vi "Acquisition_PharaGlow.vi"() -> ()   [LabVIEW 2021]
uses:
  <vilib>/userdefined/High Color/IMAQdx.ctl
  <vilib>/vision/Image Controls.llb/IMAQ Image.ctl
  <vilib>/vision/driver/IMAQdx.llb/IMAQdx Buffer Number Mode.ctl
  <vilib>/Utility/file.llb/Write Delimited Spreadsheet (string).vi
  <vilib>/Utility/file.llb/Write Delimited Spreadsheet (DBL).vi
  <vilib>/vision/driver/NI_Vision_Acquisition_Software.lvlib
  <resource>/objmgr/imaqdx.rc
  <vilib>/vision/NI_Vision_Development_Module.lvlib
panel:
  in  "Data saving folder":path=path "C:/DefaultFolder/BASLER"
  in  "Choose camera":T1="cam1"
  out "WormCounter":u64
  out "Objects":T2(array[cluster]) {"Aspect Ratio" format="%.2f"; "Orientation" format="%.2f"; "Area" format="%.2f"; "Object Center"."Y" format="%.2f"; "Object Center"."X" format="%.2f"}
  in  "Settings segmentation":T3={"Objects"=0, "Threshold"=24, "Reject Border"=TRUE, "Fill Holes"=FALSE, "Min Object Size"=TRUE, "Min Size"=300, "Max Object Size"=FALSE, "Max Size"=100, "Show Search Area"=FALSE, "Show Center"=FALSE, "Show Bounding Box"=FALSE} {"Objects" items=["Bright Objects", "Dark Objects"]; "Threshold" min=1 max=999999999 step=1; "Max Size" min=1 max=999999999 step=1; "Min Size" min=1 max=999999999 step=1}
  in  "Header Info":string[][](array[string])=[["Frame", "X_left", "Y_top", "X_center", "Y_center", "File_name"]]
  out "Path csv":path
  out "Rec_folder":path
  in  "Segment Data":bool
  out "Im_OneWorm":T4
  out "Im_Segm.":T4
  in  "Image format":string(combo)=".tiff"
  out "Init":bool
  in  "Load settings":bool
  out "Buffer overflow":string
  out "Overflow":bool=TRUE
  out "Buffer used (frames)":u64(slide) scale=0.0..167.0
  out "Expected Time (s)":dbl
  out "RAM needed (GB)":dbl
  out "Time log (ms)":dbl[](array[numeric]) format="%#_14g"
  out "Timestamp":dbl[](array[numeric])
  in  "Camera Control":T5={"Acquisition Freq"=30.0, "Exposure (ms)"=4.0, "Gain"=24.0, "Height"=2064, "Width"=3088, "Acq. trigger start"=FALSE} {"Acquisition Freq" min=1e-06 max=60.0; "Height" min=400 max=2064 step=1; "Width" min=400 max=3088 step=1}
  out "Camera Control copy":T5
  out "All Image Buffers":T4[](array[typedef])
  out "Image Out":T4(plugin-control)
  out "Lost frames":u32
  out "Approx. Frame Rate":dbl
  out "Saved frames":u32
  in  "Acquire button":bool
  in  "Focus button":bool
  out "Readout frames":i32
  in  "Stop":bool caption="Stop (F)"
  out "Finished acquisition":bool=TRUE
  in  "Num frames":u32=2000
  out "#Frames Buffer":u32=4000
  out "Camera Session":T1
  out "Camera config":string
  # "Compact data"
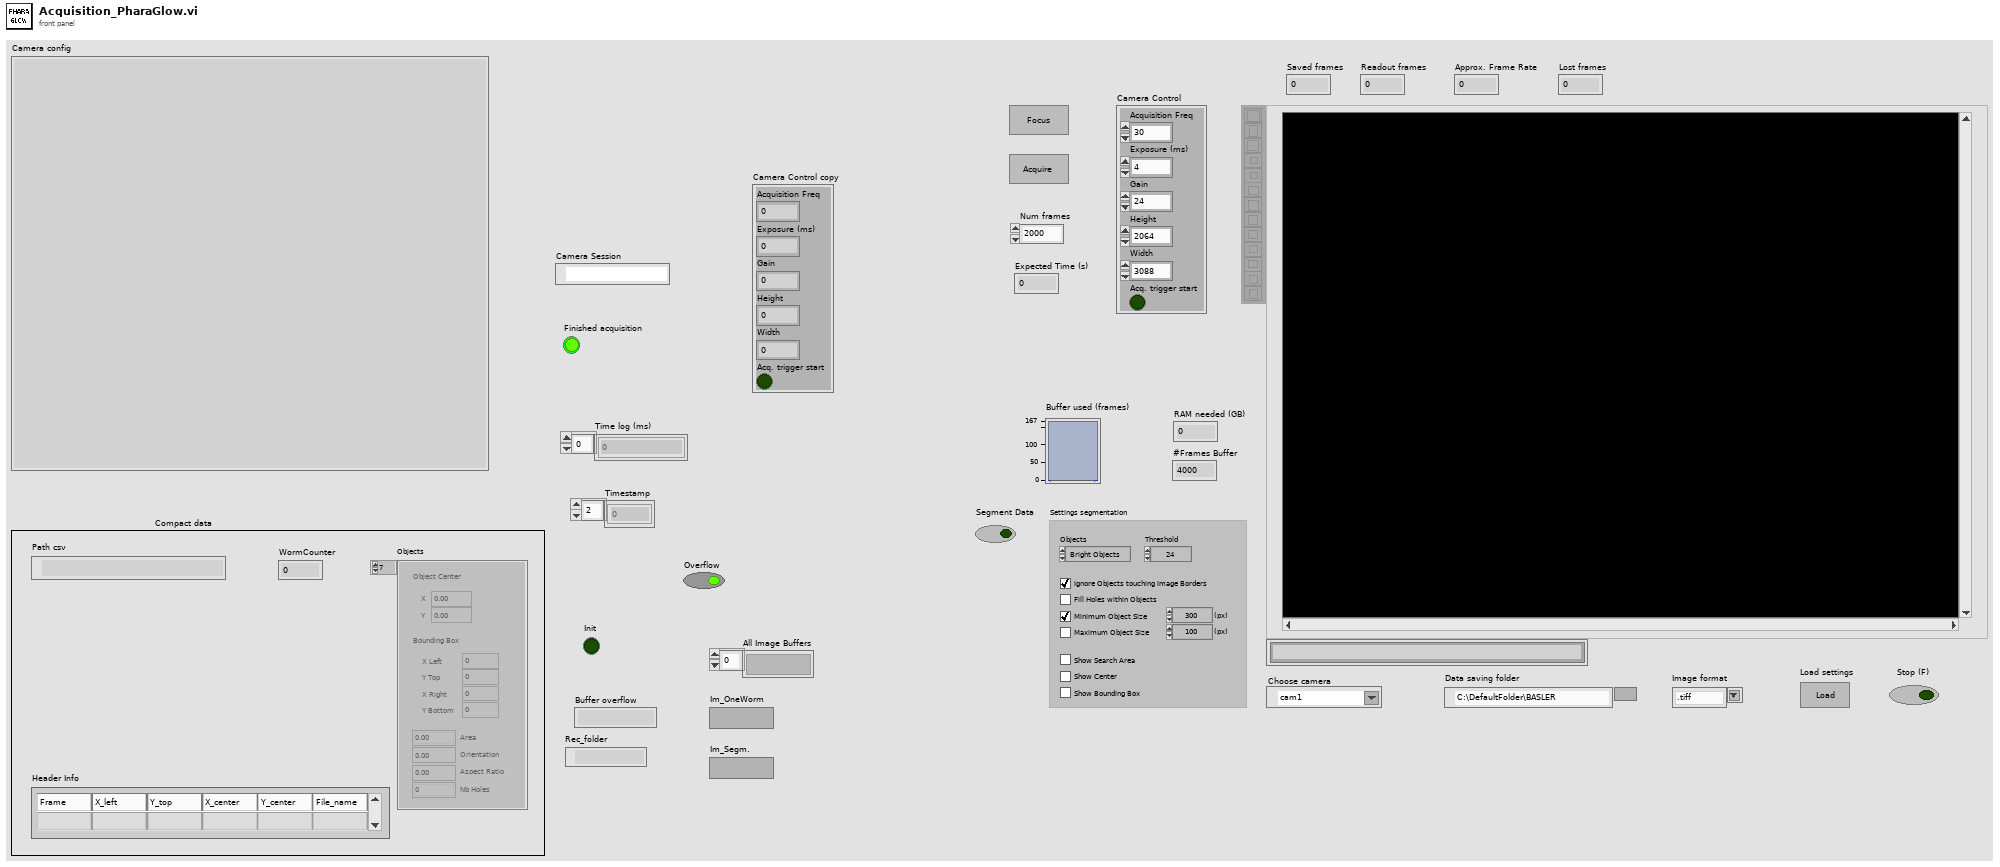
[diagram p1: front panel]
types:
  T1 = typedef "IMAQdx.ctl" = refnum<k21>
  T2 = cluster{"Object Center":cluster{"X":sgl, "Y":sgl}, "Bounding Box":cluster{"X Left":i32, "Y Top":i32, "X Right":i32, "Y Bottom":i32}, "Area":sgl, "Orientation":sgl, "Aspect Ratio":sgl, "Nb Holes":i32}[]
  T3 = cluster{"Objects":u16, "Threshold":i32, "Reject Border":bool, "Fill Holes":bool, "Min Object Size":bool, "Min Size":i32, "Max Object Size":bool, "Max Size":i32, "Show Search Area":bool, "Show Center":bool, "Show Bounding Box":bool}
  T4 = typedef "IMAQ Image.ctl" = refnum<image>
  T5 = cluster{"Acquisition Freq":dbl, "Exposure (ms)":dbl, "Gain":sgl, "Height":u16, "Width":u16, "Acq. trigger start":bool}
  T6 = enum8{"Enabled", "Disabled", "Disabled and Grayed Out"}
  T7 = typedef "NI_Vision_Acquisition_Software.lvlib/IMAQdx Buffer Number Mode.ctl" = enum32{"Next", "Last", "Buffer Number", "Every", "Last New"}
  T8 = cluster{"Acquisition Freq":bool, "Exposure (ms)":bool, "Gain":bool, "Height":bool, "Width":bool, "Acq. trigger start":bool}
  T9 = typedef "Image Type" = u32
  T10 = cluster{"X Left":i32, "Y Top":i32, "X Right":i32, "Y Bottom":i32}
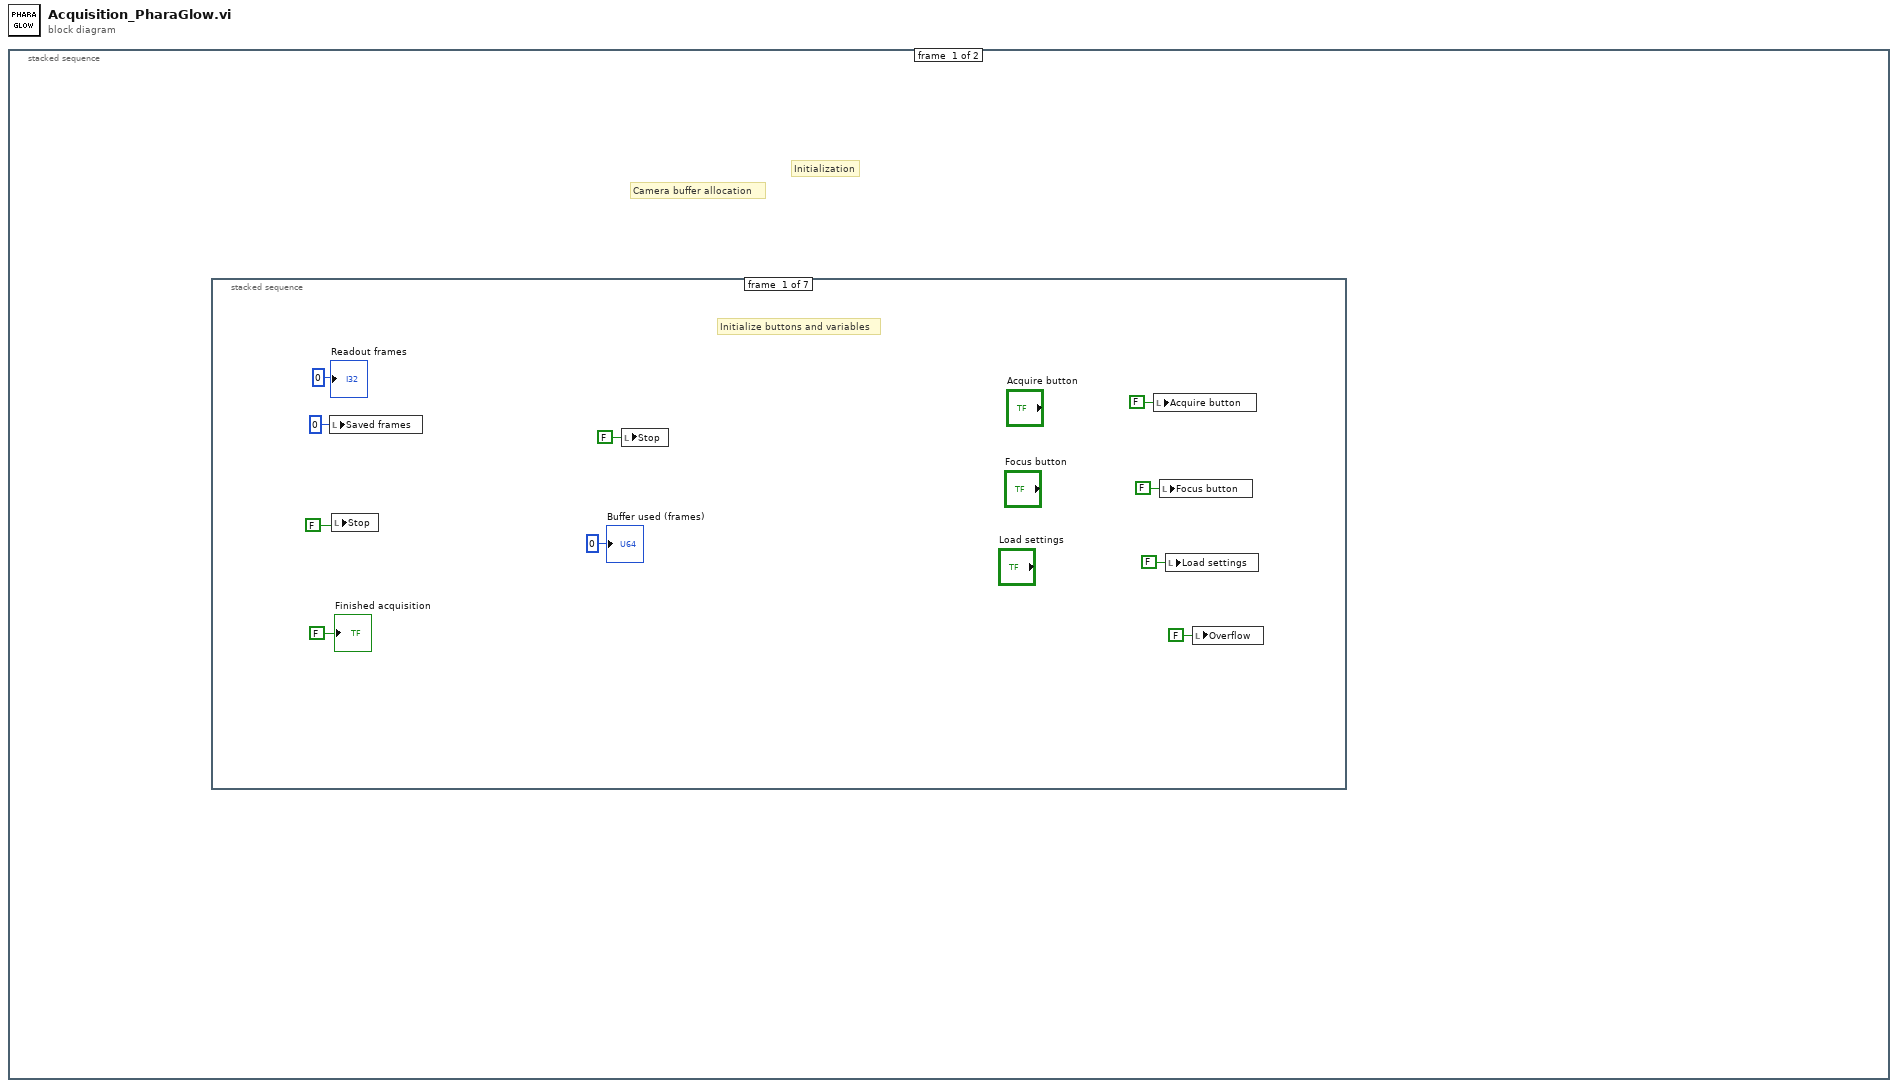
[diagram p0: block diagram]
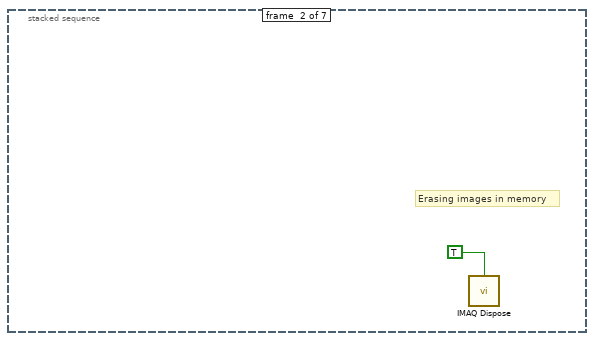
[diagram p2: hidden frame]
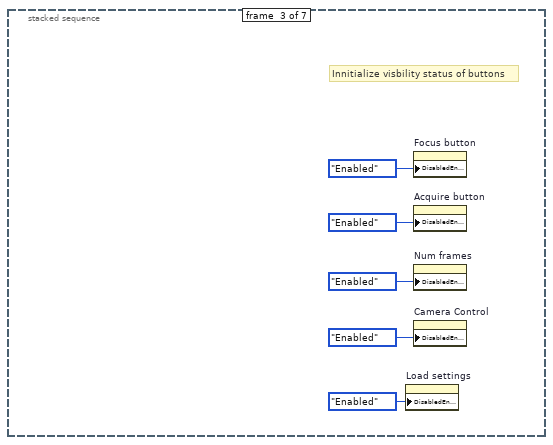
[diagram p3: hidden frame]
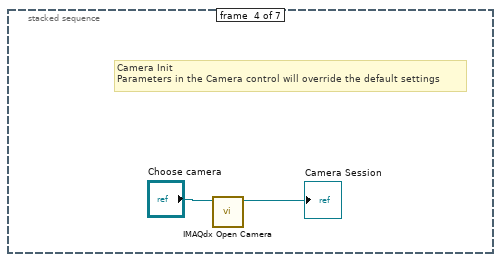
[diagram p4: hidden frame]
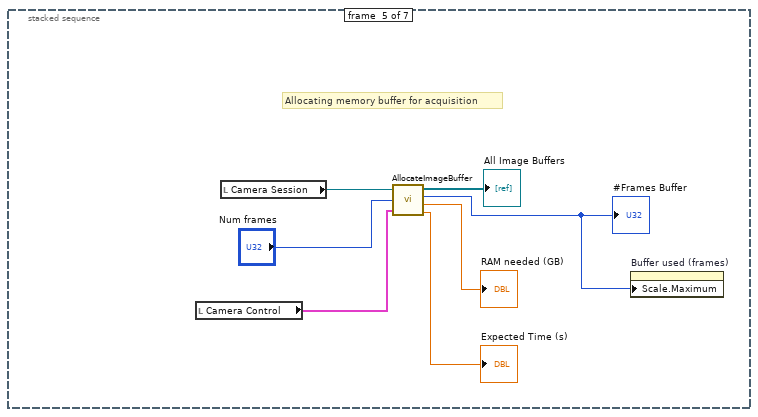
[diagram p5: hidden frame]
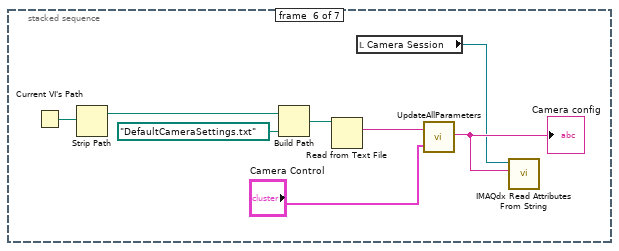
[diagram p6: hidden frame]
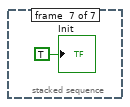
[diagram p7: hidden frame]
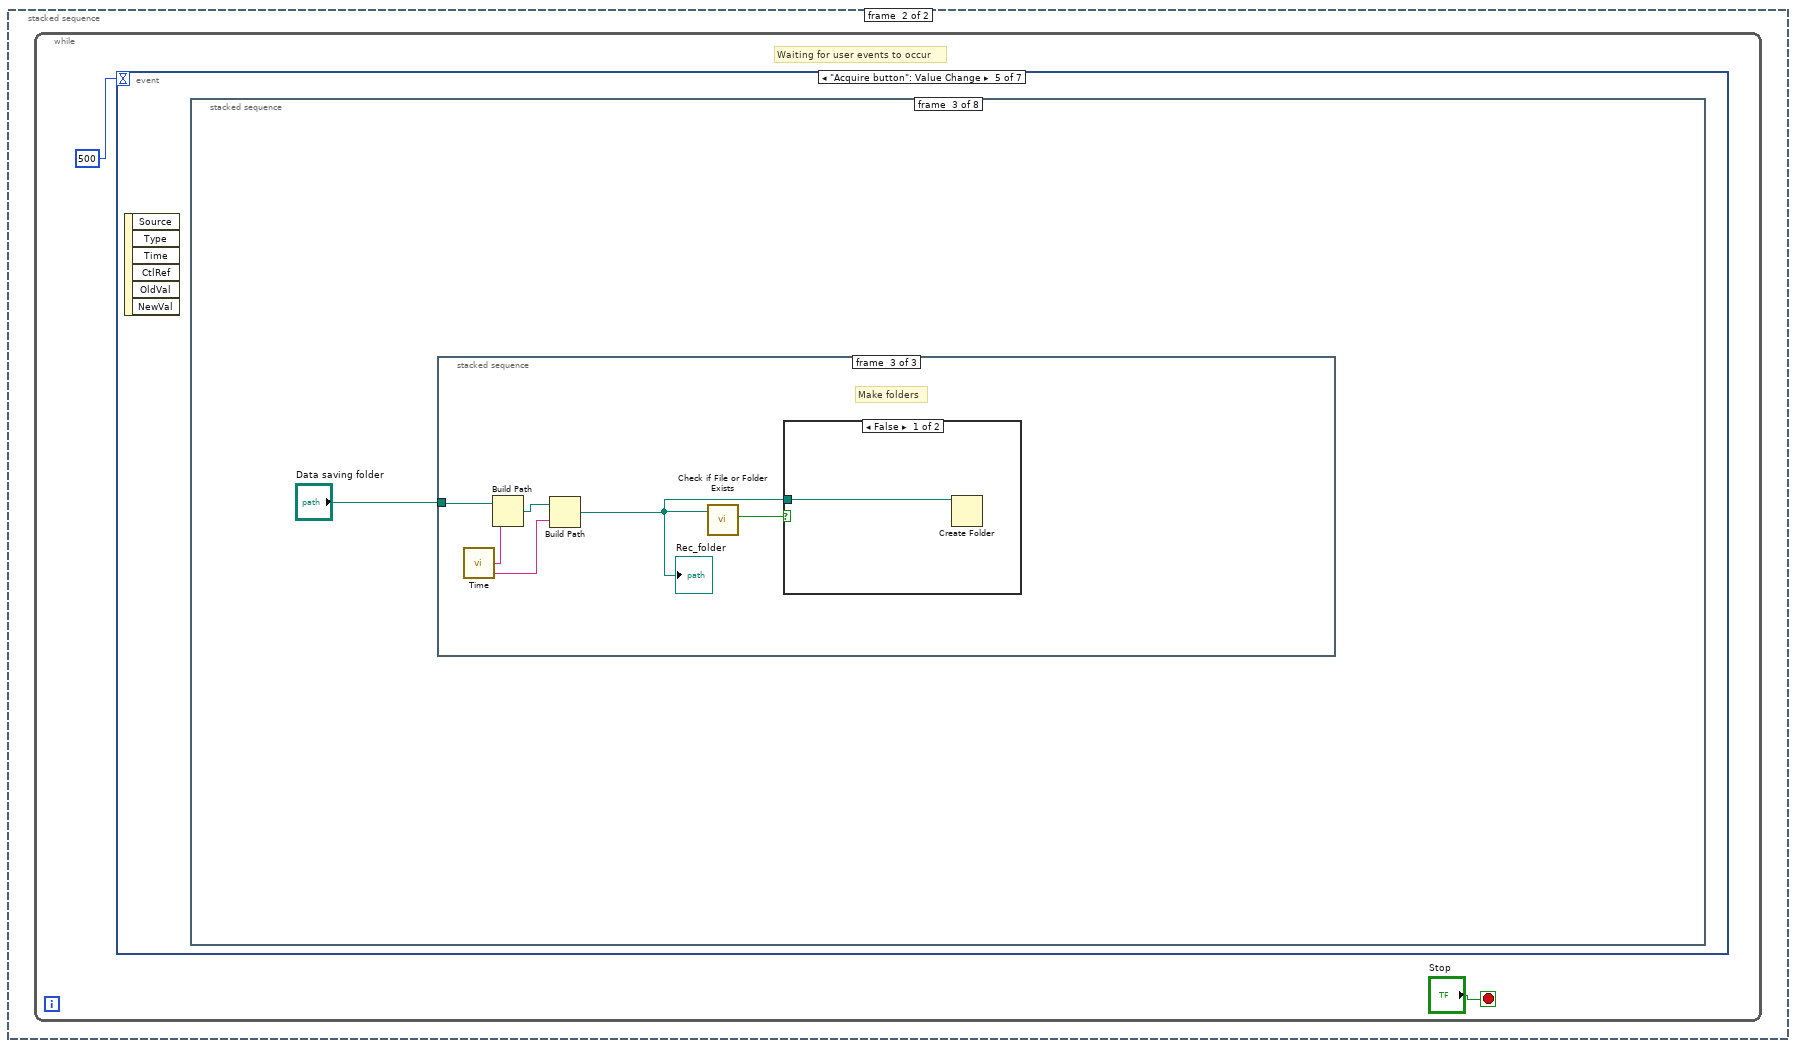
[diagram p8: hidden frame]
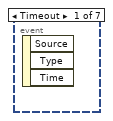
[diagram p9: hidden frame]
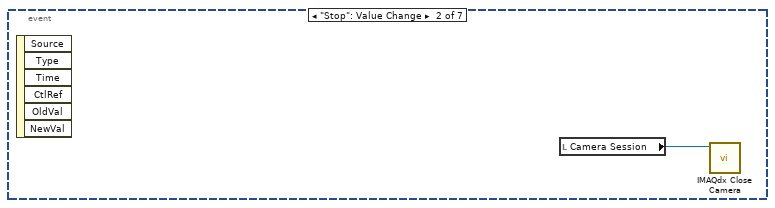
[diagram p10: hidden frame]
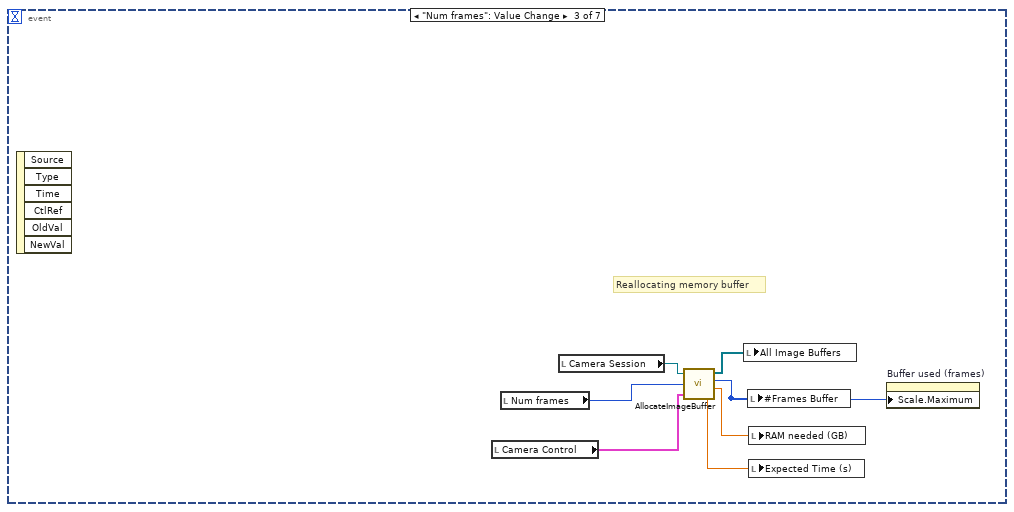
[diagram p11: hidden frame]
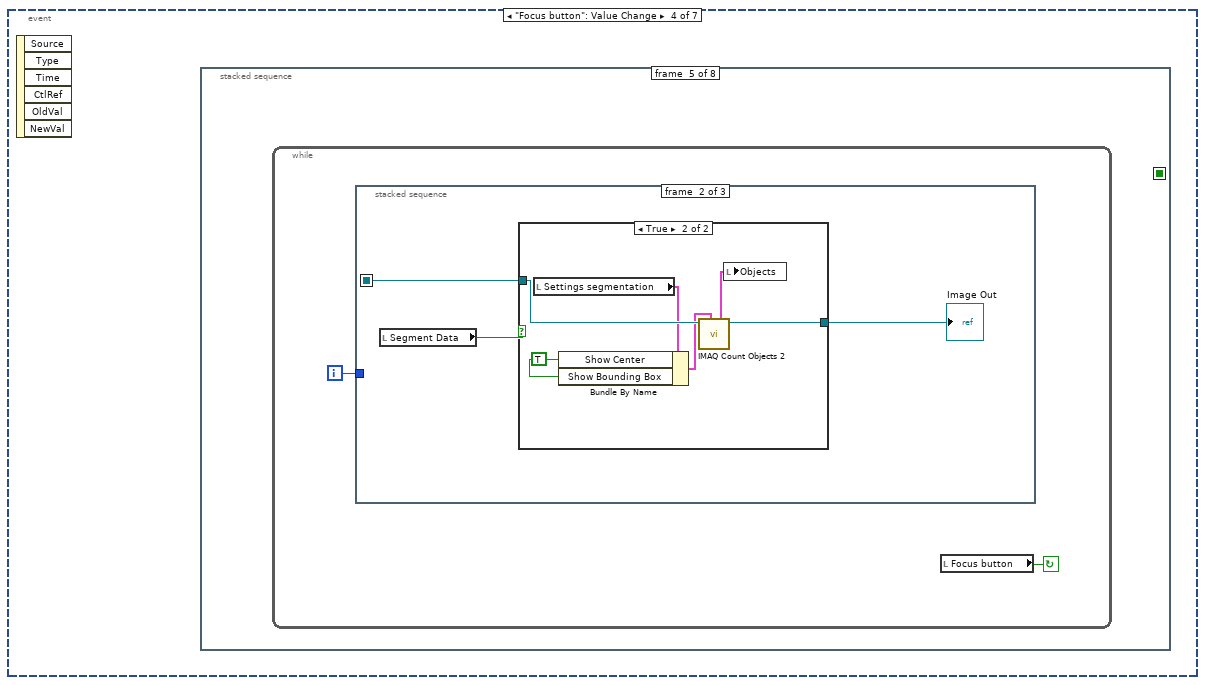
[diagram p12: hidden frame]
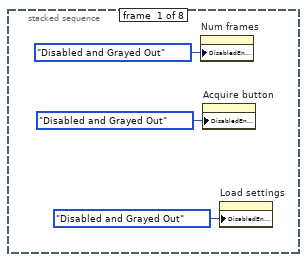
[diagram p13: hidden frame]
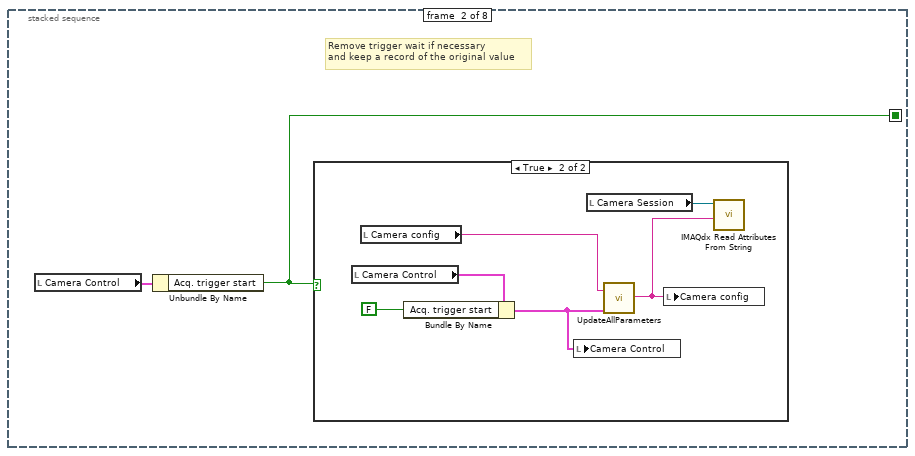
[diagram p14: hidden frame]
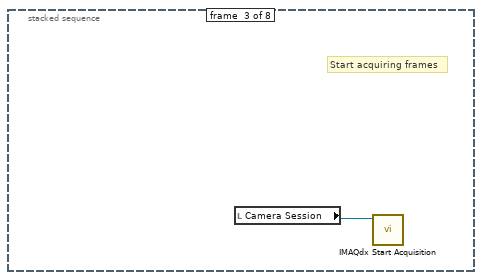
[diagram p16: hidden frame]
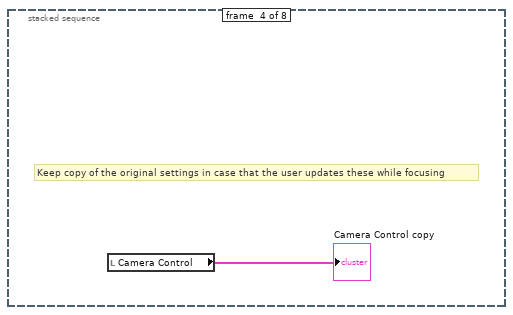
[diagram p17: hidden frame]
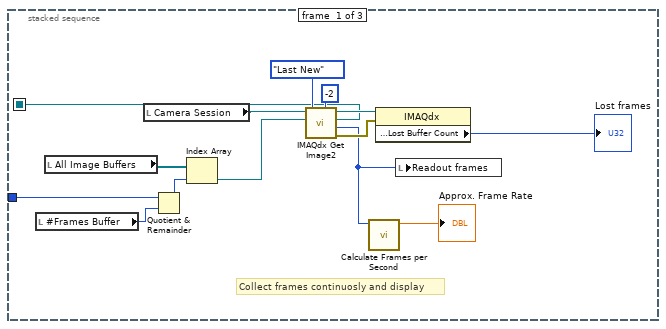
[diagram p18: hidden frame]
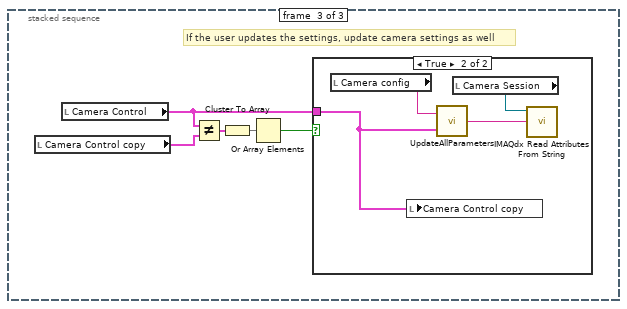
[diagram p20: hidden frame]
diagram:
  n1 = stacked-sequence {
    frame #0 {
      # "Camera buffer allocation"
      # "Initialization"
      n2 = stacked-sequence {
        frame #0 {
          # "Initialize buttons and variables"
          n3 = local write "Saved frames"(u32 0 ("Saved frames")) -> ()
          n4 = local write "Stop"(FALSE ("Stop")) -> ()
          n5 = local write "Stop"(FALSE ("Stop")) -> ()
          n6 = local write "Acquire button"(FALSE ("Acquire button")) -> ()
          n7 = local write "Focus button"(FALSE ("Focus button")) -> ()
          n8 = local write "Load settings"(FALSE ("Load settings")) -> ()
          n9 = local write "Overflow"(FALSE ("Overflow")) -> ()
          "Finished acquisition" <- FALSE
          "Readout frames" <- 0 ("Read-out frames")
          "Buffer used (frames)" <- u64 0 ("Buffer in use")
        }
        frame #1 {
          # "Erasing images in memory"
          n10 = call "IMAQ Dispose"("All Images? (No)"=TRUE) -> ()  [unwired: 5 in, 1 out]
        }
        frame #2 {
          # "Innitialize visbility status of buttons"
          n11 = property on="Load settings" class="Bool (strict)"("DisabledEnum"=T6."Enabled" ("Disabled")) -> ()  [unwired: 2 in, 2 out]
          n12 = property on="Focus button" class="Bool (strict)"("DisabledEnum"=T6."Enabled" ("Disabled")) -> ()  [unwired: 2 in, 2 out]
          n13 = property on="Acquire button" class="Bool (strict)"("DisabledEnum"=T6."Enabled" ("Disabled")) -> ()  [unwired: 2 in, 2 out]
          n14 = property on="Num frames" class="DigNum (strict)"("DisabledEnum"=T6."Enabled" ("Disabled")) -> ()  [unwired: 2 in, 2 out]
          n15 = property on="Camera Control" class="Clust (strict)"("DisabledEnum"=T6."Enabled" ("Disabled")) -> ()  [unwired: 2 in, 2 out]
        }
        frame #3 {
          # "Camera Init \nParameters in the Camera control will override the default settings"
          n16 = call <vilib>:"IMAQdx Open Camera.vi"("Session In"="Choose camera") -> ("Session Out"=→"Camera Session":T1)  [unwired: 2 in, 8 out]
        }
        frame #4 {
          # "Allocating memory buffer for acquisition"
          n17 = local read "Camera Control"() -> (w22:T5)
          n18 = local read "Camera Session"() -> (w24:T1)
          n19 = call "AllocateImageBuffer.vi"("Camera Session"=w24, "Required num frames"="Num frames", "Camera Control"=w22) -> ("All Image Buffers"=→"All Image Buffers":T4[], "#Frames Buffer"=w19:u32, "RAM Needed (GB)"=→"RAM needed (GB)":dbl, "Recording Time (s)"=→"Expected Time (s)":dbl)
          "#Frames Buffer" <- w19
          n20 = property on="Buffer used (frames)" class="Slide (strict)"("Scale.Maximum"=w19) -> ()  [unwired: 2 in, 2 out]
        }
        frame #5 {
          n21 = Current VI's Path() -> (path=w27:path)
          n22 = Strip Path(path=w27) -> (stripped path=w26:path)  [unwired: 1 out]
          n23 = Build Path(base path=w26, name or relative path=path "DefaultCameraSettings.txt") -> (appended path=w28:path)
          n24 = Read from Text File(file (use dialog)=w28) -> (text=w33:string)  [unwired: 3 in, 3 out]
          n25 = local read "Camera Session"() -> (w30:T1)
          n26 = call "UpdateAllParameters.vi"("Camera Control"="Camera Control", "Camera config in"=w33) -> ("Camera config out"=w31:string)
          "Camera config" <- w31
          n27 = call <vilib>:"IMAQdx Read Attributes From String.vi"("Attributes String In"=w31, "Session In"=w30) -> ()  [unwired: 1 in, 9 out]
        }
        frame #6 {
          "Init" <- TRUE ("Init")
        }
      }
    }
    frame #1 {
      n28 = while {
        stop <- "Stop" stop-if-true
        # "Waiting for user events to occur"
        n29 = event shown="[4] \"Acquire button\": Value Change" {
          selector: _ -> [_ _ _ _ _ _ _]
          dyn-events: _ -> [_ _ _ _ _ _ _]
          timeout: 500 -> [_ _ _ _ _ _ _]
          event Timeout {
            n30 = event-data() -> ()  [unwired: 1 in, 3 out]
          }
          event "Stop": Value Change {
            n31 = event-data() -> ()  [unwired: 1 in, 6 out]
            n32 = local read "Camera Session"() -> (w37:T1)
            n33 = call <vilib>:"IMAQdx Close Camera.vi"("Session In"=w37) -> ()  [unwired: 1 in, 10 out]
          }
          event "Num frames": Value Change {
            # "Reallocating memory buffer"
            n34 = event-data() -> ()  [unwired: 1 in, 6 out]
            n35 = local read "Camera Control"() -> (w41:T5)
            n36 = local read "Num frames"() -> (w42:u32)
            n37 = local read "Camera Session"() -> (w43:T1)
            n38 = call "AllocateImageBuffer.vi"("Camera Session"=w43, "Required num frames"=w42, "Camera Control"=w41) -> ("All Image Buffers"=w44:T4[], "#Frames Buffer"=w38:u32, "RAM Needed (GB)"=w40:dbl, "Recording Time (s)"=w39:dbl)
            n39 = local write "All Image Buffers"(w44) -> ()
            n40 = local write "#Frames Buffer"(w38) -> ()
            n41 = local write "RAM needed (GB)"(w40) -> ()
            n42 = local write "Expected Time (s)"(w39) -> ()
            n43 = property on="Buffer used (frames)" class="Slide (strict)"("Scale.Maximum"=w38) -> ()  [unwired: 2 in, 2 out]
          }
          event "Focus button": Value Change {
            n44 = event-data() -> ()  [unwired: 1 in, 6 out]
            n45 = stacked-sequence {
              seq-local: [_ w48 _ _ _ _ _ _] -> [_ _ _ _ _ _ w98 _]
              frame #0 {
                n46 = property on="Num frames" class="DigNum (strict)"("DisabledEnum"=T6."Disabled and Grayed Out" ("Disabled")) -> ()  [unwired: 2 in, 2 out]
                n47 = property on="Acquire button" class="Bool (strict)"("DisabledEnum"=T6."Disabled and Grayed Out" ("Disabled")) -> ()  [unwired: 2 in, 2 out]
                n48 = property on="Load settings" class="Bool (strict)"("DisabledEnum"=T6."Disabled and Grayed Out" ("Disabled")) -> ()  [unwired: 2 in, 2 out]
              }
              frame #1 {
                # "Remove trigger wait if necessary\nand keep a record of the original value"
                n49 = local read "Camera Control"() -> (w49:T5)
                n50 = Unbundle By Name(w49) -> ("Acq. trigger start"=w48:bool)
                n51 = case shown="True" w48 {
                  frame False {
                  }
                  frame True {
                    n52 = local read "Camera Control"() -> (w55:T5)
                    n53 = local read "Camera config"() -> (w53:string)
                    n54 = Bundle By Name(cluster=w55, "Acq. trigger start"=FALSE ("Acquisition trigger start")) -> (w50:T5)
                    n55 = local write "Camera Control"(w50) -> ()
                    n56 = local read "Camera Session"() -> (w52:T1)
                    n57 = call "UpdateAllParameters.vi"("Camera Control"=w50, "Camera config in"=w53) -> ("Camera config out"=w51:string)
                    n58 = local write "Camera config"(w51) -> ()
                    n59 = call <vilib>:"IMAQdx Read Attributes From String.vi"("Attributes String In"=w51, "Session In"=w52) -> ()  [unwired: 1 in, 9 out]
                  }
                }
              }
              frame #2 {
                # "Start acquiring frames"
                n60 = local read "Camera Session"() -> (w56:T1)
                n61 = call <vilib>:"IMAQdx Start Acquisition.vi"("Session In"=w56) -> ()  [unwired: 1 in, 10 out]
              }
              frame #3 {
                # "Keep copy of the original settings in case that the user updates these while focusing"
                n62 = local read "Camera Control"() -> (→"Camera Control copy":T5)
              }
              frame #4 {
                n63 = while {
                  i -> [w58]
                  stop <- w59 continue-if-true
                  n64 = stacked-sequence {
                    seq-local: [w60 _ _] -> [_ w75 _]
                    tunnel: w58 -> [w61 _ _]
                    frame #0 {
                      # "Collect frames continuosly and display"
                      n65 = local read "#Frames Buffer"() -> (w66:u32)
                      n66 = local read "All Image Buffers"() -> (w68:T4[])
                      n67 = local read "Camera Session"() -> (w69:T1)
                      n68 = Quotient & Remainder(x=w61, y=w66) -> (x-y*floor(x/y)=w65:u32)  [unwired: 1 out]
                      n69 = Index Array(array=w68, index=w65) -> (element=w67:T4)
                      n70 = call <vilib>:"IMAQdx Get Image2.vi"("Timeout (ms)"=-2, "Buffer Number Mode (Next)"=IMAQdx_Buffer_Number_Mode."Last New", "Image In"=w67, "Session In"=w69) -> ("error out"=w72:errorcluster, "Buffer Number Out"=w62:u32, "Image Out"=w60:T4, "Session Out"=w73:T1)  [unwired: 4 in]
                      n71 = call <vilib>:"Calculate Frames per Second.vi"("Buffer Number"=w62) -> ("Acquired Frames/s"=→"Approx. Frame Rate":dbl)  [unwired: 2 in, 8 out]
                      n72 = property class="IMAQdx"(reference=w73, error in=w72) -> ("Status Information:Lost Buffer Count"=→"Lost frames":u32)  [unwired: 2 out]
                      n73 = local write "Readout frames"(w62) -> ()
                    }
                    frame #1 {
                      n74 = local read "Segment Data"() -> (w76:bool)
                      n75 = case shown="True" w76 {
                        tunnel: w75 -> [w77 w82]
                        tunnel: [w77 w81] -> w74
                        frame False {
                        }
                        frame True {
                          w79 = TRUE ("Show Center")
                          n76 = local read "Settings segmentation"() -> (w80:T3)
                          n77 = Bundle By Name(cluster=w80, "Show Center"=w79, "Show Bounding Box"=w79) -> (w78:T3)
                          n78 = call "IMAQ Count Objects 2"("Settings"=w78, "Image"=w82) -> ("Image Out"=w81:T4, "Objects"=w83:T2)  [unwired: 5 in, 3 out]
                          n79 = local write "Objects"(w83) -> ()
                        }
                      }
                      "Image Out" <- w74
                    }
                    frame #2 {
                      # "If the user updates the settings, update camera settings as well"
                      n80 = local read "Camera Control copy"() -> (w84:T5)
                      n81 = local read "Camera Control"() -> (w85:T5)
                      n82 = Not Equal?(x=w85, y=w84) -> (x != y?=w88:T8)
                      n83 = Cluster To Array(cluster=w88) -> (array=w87:bool[])
                      n84 = Or Array Elements(Boolean array=w87) -> (logical OR=w86:bool)
                      n85 = case shown="True" w86 {
                        tunnel: w85 -> [_ w89]
                        frame False {
                        }
                        frame True {
                          n86 = local read "Camera config"() -> (w92:string)
                          n87 = local write "Camera Control copy"(w89) -> ()
                          n88 = call "UpdateAllParameters.vi"("Camera Control"=w89, "Camera config in"=w92) -> ("Camera config out"=w91:string)
                          n89 = local read "Camera Session"() -> (w90:T1)
                          n90 = call <vilib>:"IMAQdx Read Attributes From String.vi"("Attributes String In"=w91, "Session In"=w90) -> ()  [unwired: 1 in, 9 out]
                        }
                      }
                    }
                  }
                  n91 = local read "Focus button"() -> (w59:bool)
                }
              }
              frame #5 {
                n92 = local read "Camera Session"() -> (w93:T1)
                n93 = call <vilib>:"IMAQdx Stop Acquisition.vi"("Session In"=w93) -> ()  [unwired: 9 in, 2 out]
              }
              frame #6 {
                # "Recover original settings for the trigger"
                n94 = local read "Camera Control"() -> (w99:T5)
                n95 = Bundle By Name(cluster=w99, "Acq. trigger start"=w98) -> (w96:T5)
                n96 = local read "Camera config"() -> (w97:string)
                n97 = local write "Camera Control"(w96) -> ()
                n98 = call "UpdateAllParameters.vi"("Camera Control"=w96, "Camera config in"=w97) -> ("Camera config out"=w94:string)
                n99 = local read "Camera Session"() -> (w95:T1)
                n100 = local write "Camera config"(w94) -> ()
                n101 = call <vilib>:"IMAQdx Read Attributes From String.vi"("Attributes String In"=w94, "Session In"=w95) -> ()  [unwired: 1 in, 9 out]
              }
              frame #7 {
                n102 = local write "Focus button"(FALSE ("Focus button")) -> ()
                n103 = property on="Acquire button" class="Bool (strict)"("DisabledEnum"=T6."Enabled" ("Disabled")) -> ()  [unwired: 2 in, 2 out]
                n104 = property on="Num frames" class="DigNum (strict)"("DisabledEnum"=T6."Enabled" ("Disabled")) -> ()  [unwired: 2 in, 2 out]
                n105 = property on="Load settings" class="Bool (strict)"("DisabledEnum"=T6."Enabled" ("Disabled")) -> ()  [unwired: 2 in, 2 out]
              }
            }
          }
          event "Acquire button": Value Change {
            n106 = event-data() -> ()  [unwired: 1 in, 6 out]
            n107 = stacked-sequence {
              frame #0 {
                n108 = property on="Load settings" class="Bool (strict)"("DisabledEnum"=T6."Disabled and Grayed Out" ("Disabled")) -> ()  [unwired: 2 in, 2 out]
                n109 = property on="Camera Control" class="Clust (strict)"("DisabledEnum"=T6."Disabled and Grayed Out" ("Disabled")) -> ()  [unwired: 2 in, 2 out]
                n110 = property on="Focus button" class="Bool (strict)"("DisabledEnum"=T6."Disabled and Grayed Out" ("Disabled")) -> ()  [unwired: 2 in, 2 out]
              }
              frame #1 {
                # "Here camera aquires"
                n111 = local read "Camera Session"() -> (w112:T1)
                n112 = local read "Camera Control"() -> (w110:T5)
                n113 = local read "Camera config"() -> (w111:string)
                n114 = call "UpdateAllParameters.vi"("Camera Control"=w110, "Camera config in"=w111) -> ("Camera config out"=w109:string)
                n115 = call <vilib>:"IMAQdx Read Attributes From String.vi"("Attributes String In"=w109, "Session In"=w112) -> ("error out"=w107:errorcluster, "Session Out"=w108:T1)  [unwired: 1 in, 7 out]
                n116 = call <vilib>:"IMAQdx Start Acquisition.vi"("error in"=w107, "Session In"=w108) -> ()  [unwired: 10 out]
              }
              frame #2 {
                n117 = stacked-sequence {
                  tunnel: "Data saving folder" -> [_ w119 w126]
                  frame #0 {
                    # "resetting counter of frames saved"
                    # "Waiting time to ensure that acquisition is already on its way and that frames are waiting in the buffer"
                    n118 = local write "Saved frames"(0 ("Saved images")) -> ()
                    n119 = Wait (ms)(milliseconds to wait=u32 100) -> ()  [unwired: 1 out]
                  }
                  frame #1 {
                    # "Make folders"
                    n120 = call "Time.vi"() -> ("Date"=w118:string)  [unwired: 2 out]
                    n121 = Build Path(base path=w119, name or relative path=w118) -> (appended path=w116:path)
                    n122 = call <vilib>:"Check if File or Folder Exists.vi"("path"=w116) -> ("file or folder exists?"=w117:bool)  [unwired: 8 in, 2 out]
                    n123 = case shown="True" w117 {
                      tunnel: w116 -> [w120 _]
                      frame False {
                        n124 = Create Folder(path (use dialog)=w120) -> ()  [unwired: 2 in, 3 out]
                      }
                      frame True {
                      }
                    }
                  }
                  frame #2 {
                    # "Make folders"
                    n125 = call "Time.vi"() -> ("Time"=w122:string, "Date"=w124:string)  [unwired: 1 out]
                    n126 = Build Path(base path=w126, name or relative path=w124) -> (appended path=w123:path)
                    n127 = Build Path(base path=w123, name or relative path=w122) -> (appended path=w121:path)
                    "Rec_folder" <- w121
                    n128 = call <vilib>:"Check if File or Folder Exists.vi"("path"=w121) -> ("file or folder exists?"=w125:bool)  [unwired: 8 in, 2 out]
                    n129 = case shown="False" w125 {
                      tunnel: w121 -> [w127 _]
                      frame False {
                        n130 = Create Folder(path (use dialog)=w127) -> ()  [unwired: 2 in, 3 out]
                      }
                      frame True {
                      }
                    }
                  }
                }
              }
              frame #3 {
                # "Prepare the system for the compact data option\nwhere only the single segmented worms are saved\nI will pressume that we use 8-bit data"
                n131 = case shown="True" "Segment Data" {
                  frame False {
                  }
                  frame True {
                    n132 = stacked-sequence {
                      frame #0 {
                        w130 = T9 0 items=["Grayscale (U8)", "Grayscale (I16)", "Grayscale (SGL)", "Complex (CSG)", "RGB (U32)", "HSL (U32)", "RGB (U64)", "Grayscale (U16)"] ("Image Type")
                        w131 = T9 0 items=["Grayscale (U8)", "Grayscale (I16)", "Grayscale (SGL)", "Complex (CSG)", "RGB (U32)", "HSL (U32)", "RGB (U64)", "Grayscale (U16)"] ("Image Type")
                        n133 = call "IMAQ Create"("Image Name"="Segmentation", "Image Type"=w130) -> ("New Image"=→"Im_Segm.":T4)  [unwired: 3 in, 1 out]
                        n134 = call "IMAQ Create"("Image Name"="WormBox", "Image Type"=w131) -> ("New Image"=→"Im_OneWorm":T4)  [unwired: 3 in, 1 out]
                        "WormCounter" <- u64 0
                      }
                      frame #1 {
                        n135 = local read "Rec_folder"() -> (w139:path)
                        n136 = Build Path(base path=w139, name or relative path="Coordinates.csv") -> (appended path=w142:path)
                        n137 = call-poly <vilib>:"Write Delimited Spreadsheet.vi"("file path (dialog if empty)"=w142, "2D data"="Header Info", "append to file? (new file:F)"=FALSE, "delimiter (\\t)"="," ("delimiter (\\t)")) -> ("new file path (Not A Path if cancelled)"=→"Path csv":path)  [unwired: 10 in, 1 out]
                      }
                    }
                  }
                }
              }
              frame #4 {
                # "Save images in parallel"
                # "Collect frames continuosly and display"
                n138 = while {
                  tunnel: [w262] -> w143 mode=indexing
                  tunnel: [TRUE] -> w144
                  i -> [w267]
                  stop <- w265 stop-if-true
                  n139 = local read "#Frames Buffer"() -> (w253:u32)
                  n140 = local read "All Image Buffers"() -> (w255:T4[])
                  n141 = local read "Settings segmentation"() -> (w245:T3)
                  n142 = local read "Camera Session"() -> (w256:T1)
                  n143 = Quotient & Remainder(x=w267, y=w253) -> (x-y*floor(x/y)=w252:u32)  [unwired: 1 out]
                  n144 = Index Array(array=w255, index=w252) -> (element=w254:T4)
                  n145 = Unbundle By Name(w245) -> ("Show Bounding Box"=w244:bool)
                  n146 = call <vilib>:"IMAQdx Get Image2.vi"("Timeout (ms)"=-2, "Buffer Number Mode (Next)"=IMAQdx_Buffer_Number_Mode."Every", "Image In"=w254, "Session In"=w256) -> ("error out"=w259:errorcluster, "Buffer Number Out"=w248:u32, "Image Out"=w246:T4, "Session Out"=w247:T1)  [unwired: 4 in]
                  n147 = local read "Segment Data"() -> (w243:bool)
                  n148 = Increment(x=w248) -> (x+1=w249:u32)
                  n149 = property class="IMAQdx"(reference=w247, error in=w259) -> ("Status Information:Lost Buffer Count"=w251:u32)  [unwired: 2 out]
                  n150 = call <vilib>:"Calculate Frames per Second.vi"("Buffer Number"=w248) -> ("Acquired Frames/s"=w250:dbl)  [unwired: 2 in, 8 out]
                  n151 = local write "Approx. Frame Rate"(w250) -> ()
                  n152 = And(x=w243, y=w244) -> (x .and. y?=w242:bool)
                  n153 = local write "Readout frames"(w249) -> ()
                  n154 = local read "Num frames"() -> (w264:u32)
                  n155 = local write "Lost frames"(w251) -> ()
                  n156 = call "GetTimeStamp.vi"("Image"=w246) -> ("Time(ms)"=w262:dbl)  [unwired: 1 in, 3 out]
                  n157 = local read "Stop"() -> (w263:bool)
                  n158 = case shown="False" w242 {
                    tunnel: w246 -> [w268 _]
                    frame False {
                      n159 = local write "Image Out"(w268) -> ()
                    }
                    frame True {
                    }
                  }
                  n160 = Equal?(x=w249, y=w264) -> (x = y?=w266:bool)
                  n161 = Or(x=w266, y=w263) -> (x .or. y?=w265:bool)
                  n162 = Wait (ms)(milliseconds to wait=u32 15) -> ()  [unwired: 1 out]
                }
                "Timestamp" <- w143
                n163 = stacked-sequence {
                  frame #0 {
                    # "resetting counter of frames saved"
                    # "Waiting time to ensure that acquisition is already on its way and that frames are waiting in the buffer"
                    n164 = local write "Saved frames"(0 ("Saved images")) -> ()
                    n165 = Wait (ms)(milliseconds to wait=u32 100) -> ()  [unwired: 1 out]
                  }
                  frame #1 {
                    n166 = while {
                      stop <- w149 continue-if-true
                      n167 = local read "Finished acquisition"() -> (w150:bool)
                      n168 = local read "Saved frames"() -> (w151:u32)
                      n169 = local read "Readout frames"() -> (w152:i32)
                      n170 = Not(x=w150) -> (.not. x?=w148:bool)
                      n171 = Greater?(x=w152, y=w151) -> (0:w147:bool)
                      n172 = Or(x=w147, y=w148) -> (x .or. y?=w149:bool)
                      n173 = case shown="True" w147 {
                        frame False {
                        }
                        frame True {
                          n174 = stacked-sequence {
                            frame #0 {
                              n175 = local read "Segment Data"() -> (w154:bool)
                              n176 = local read "Saved frames"() -> (w153:u32)
                              n177 = case shown="True" w154 {
                                tunnel: w153 -> [_ w172]
                                frame False {
                                n178 = local read "#Frames Buffer"() -> (w155:u32)
                                n179 = local read "Saved frames"() -> (w159:u32)
                                n180 = local read "All Image Buffers"() -> (w166:T4[])
                                n181 = Quotient & Remainder(x=w159, y=w155) -> (x-y*floor(x/y)=w161:u32)  [unwired: 1 out]
                                n182 = Increment(x=w159) -> (x+1=w160:u32)
                                n183 = property on="Image format" class="CmbBox"() -> ("Value"=w156:string)  [unwired: 2 in, 2 out]
                                n184 = local read "Rec_folder"() -> (w158:path)
                                n185 = Number To Decimal String(number=w160) -> (decimal integer string=w164:string)  [unwired: 1 in]
                                n186 = Concatenate Strings(w164, w156) -> (w163:string)
                                n187 = Index Array(array=w166, index=w161) -> (element=w165:T4)
                                n188 = Build Path(base path=w158, name or relative path=w163) -> (appended path=w162:path)
                                n189 = case shown="\".tiff\", Default" "Image format" {
                                tunnel: w165 -> [w169 w171]
                                tunnel: w162 -> [w168 w170]
                                frame ".jpeg" {
                                n190 = call-poly "IMAQ Write File 2"("Image Quality"=u32 850, "File Path"=w168, "Image"=w169) -> ()  [unwired: 7 in, 2 out]
                                }
                                frame ".tiff", Default {
                                n191 = call-poly "IMAQ Write File 2"("File Path"=w170, "Image"=w171) -> ()  [unwired: 8 in, 2 out]
                                }
                                }
                                }
                                frame True {
                                n192 = stacked-sequence {
                                seq-local: [w173 _] -> [_ w184]
                                tunnel: w172 -> [_ w183]
                                frame #0 {
                                n193 = local read "#Frames Buffer"() -> (w179:u32)
                                n194 = local read "All Image Buffers"() -> (w181:T4[])
                                n195 = local read "Saved frames"() -> (w180:u32)
                                n196 = Quotient & Remainder(x=w180, y=w179) -> (x-y*floor(x/y)=w178:u32)  [unwired: 1 out]
                                n197 = Index Array(array=w181, index=w178) -> (element=w176:T4)
                                n198 = call "IMAQ Count Objects 2"("Settings"="Settings segmentation", "Image"=w176) -> ("Image Out"=w173:T4, "Objects"=→"Objects":T2)  [unwired: 5 in, 3 out]
                                n199 = Unbundle By Name("Settings segmentation") -> ("Show Bounding Box"=w174:bool)
                                n200 = case shown="True" w174 {
                                tunnel: w173 -> [_ w182]
                                frame False {
                                }
                                frame True {
                                n201 = local write "Image Out"(w182) -> ()
                                }
                                }
                                }
                                frame #1 {
                                n202 = local read "Im_OneWorm"() -> (w186:T4)
                                n203 = local read "Objects"() -> (w187:T2)
                                n204 = local read "Path csv"() -> (w185:path)
                                n205 = for {
                                tunnel: w184 -> [w192]
                                tunnel: w185 -> [w204]
                                tunnel: w187 -> [w198] mode=indexing
                                tunnel: w183 -> [w191]
                                shift-right: [w188] -> _
                                shift-left: w186 -> [w188]
                                n206 = Unbundle By Name(w198) -> ("Bounding Box.X Left"=w202:i32, "Bounding Box.Y Top"=w201:i32, "Object Center.X"=w200:sgl, "Object Center.Y"=w199:sgl, "Bounding Box"=w203:T10)
                                n207 = local read "WormCounter"() -> (w189:u64)
                                n208 = Increment(x=w189) -> (x+1=w190:u64)
                                n209 = local write "WormCounter"(w190) -> ()
                                n210 = Cluster To Array(cluster=w203) -> (array=w210:i32[])
                                n211 = call "IMAQ Extract 2"("Optional Rectangle"=w210, "Image Dst"=w188, "Image Src"=w192) -> ("Image Dst Out"=w193:T4)  [unwired: 7 in, 1 out]
                                n212 = Number To Decimal String(number=w189) -> (decimal integer string=w209:string)  [unwired: 1 in]
                                n213 = property on="Image format" class="CmbBox"() -> ("Value"=w196:string)  [unwired: 2 in, 2 out]
                                n214 = Build Array(w191, w202, w201, w200, w199, w189) -> (w206:sgl[])
                                n215 = local read "Rec_folder"() -> (w197:path)
                                n216 = Concatenate Strings(w209, w196) -> (w208:string)
                                n217 = call-poly <vilib>:"Write Delimited Spreadsheet.vi"("file path (dialog if empty)"=w204, "1D data"=w206, "append to file? (new file:F)"=TRUE, "delimiter (\\t)"="," ("delimiter (\\t)")) -> ()  [unwired: 10 in, 2 out]
                                n218 = Build Path(base path=w197, name or relative path=w208) -> (appended path=w195:path)
                                n219 = local read "Image format"() -> (w194:string)
                                n220 = case shown="\".tiff\", Default" w194 {
                                tunnel: w193 -> [w213 w215]
                                tunnel: w195 -> [w212 w214]
                                frame ".jpeg" {
                                n221 = call-poly "IMAQ Write File 2"("Image Quality"=u32 850, "File Path"=w212, "Image"=w213) -> ()  [unwired: 7 in, 2 out]
                                }
                                frame ".tiff", Default {
                                n222 = call-poly "IMAQ Write File 2"("File Path"=w214, "Image"=w215) -> ()  [unwired: 8 in, 2 out]
                                }
                                }
                                }
                                }
                                }
                                }
                              }
                            }
                            frame #1 {
                              n223 = local read "Saved frames"() -> (w217:u32)
                              n224 = Increment(x=w217) -> (x+1=→"Saved frames":u32)
                            }
                            frame #2 {
                              n225 = local read "Readout frames"() -> (w220:i32)
                              n226 = local read "Saved frames"() -> (w219:u32)
                              n227 = Subtract(x=w220, y=w219) -> (x-y=w218:u32)
                              n228 = local write "Buffer used (frames)"(w218) -> ()
                            }
                          }
                        }
                      }
                    }
                  }
                  frame #2 {
                    n229 = local read "Timestamp"() -> (w222:dbl[])
                    n230 = Index Array(array=w222, index=0) -> (element=w226:dbl)
                    n231 = Subtract(x=w222, y=w226) -> (x-y=w227:dbl[])
                    "Time log (ms)" <- w227
                    n232 = local read "Rec_folder"() -> (w223:path)
                    n233 = Build Path(base path=w223, name or relative path="TimeStamp.txt") -> (appended path=w228:path)
                    n234 = call-poly <vilib>:"Write Delimited Spreadsheet.vi"("file path (dialog if empty)"=w228, "1D data"=w227, "transpose? (no:F)"=TRUE) -> ()  [unwired: 11 in, 2 out]
                  }
                  frame #3 {
                    n235 = local write "Finished acquisition"(FALSE) -> ()
                  }
                }
                n236 = flat-sequence {
                  tunnel: w143 -> [_]
                  frame #0 {
                    n237 = local read "#Frames Buffer"() -> (w238:u32)
                    n238 = local read "Saved frames"() -> (w237:u32)
                    n239 = local read "Readout frames"() -> (w236:i32)
                    n240 = Number To Decimal String(number=w237) -> (decimal integer string=w232:string)  [unwired: 1 in]
                    n241 = Increment(x=w236) -> (x+1=w230:i32)
                    n242 = Add(x=w238, y=w237) -> (x+y=w235:u32)
                    n243 = Concatenate Strings("Buffer overflow at frame:" ("string"), w232) -> (w233:string)
                    "Buffer overflow" <- w233
                    n244 = Less?(x=w235, y=w230) -> (x < y?=w234:bool)
                    n245 = case shown="True" w234 {
                      tunnel: w233 -> [_ w241]
                      frame False {
                        n246 = local write "Overflow"(FALSE ("Overflow")) -> ()
                      }
                      frame True {
                        n247 = One Button Dialog(message=w241) -> ()  [unwired: 1 in, 1 out]
                        "Overflow" <- TRUE
                      }
                    }
                  }
                }
                n248 = local write "Finished acquisition"(w144) -> ()
              }
              frame #5 {
                # "Stop acquisition"
                n249 = local read "Camera Session"() -> (w269:T1)
                n250 = call <vilib>:"IMAQdx Stop Acquisition.vi"("Session In"=w269) -> ()  [unwired: 9 in, 2 out]
              }
              frame #6 {
                # "Saving settings"
                n251 = stacked-sequence {
                  seq-local: [_ w274 _] -> [_ _ w280]
                  frame #0 {
                    # "Save camera settings"
                    n252 = local read "Rec_folder"() -> (w272:path)
                    n253 = local read "Camera config"() -> (w270:string)
                    n254 = Build Path(base path=w272, name or relative path="CameraSettings.txt") -> (appended path=w271:path)
                    n255 = Write to Text File(file (use dialog)=w271, text=w270) -> ()  [unwired: 2 in, 3 out]
                  }
                  frame #1 {
                    # "Gathering additional Info"
                    n256 = local read "Overflow"() -> (w277:bool)
                    n257 = case shown="True" w277 {
                      tunnel: ["No overflow" w279] -> w275
                      frame False {
                      }
                      frame True {
                        n258 = local read "Buffer overflow"() -> (w279:string)
                      }
                    }
                    n259 = Concatenate Strings("", w275) -> (w274:string)
                  }
                  frame #2 {
                    # "Save additional information"
                    n260 = local read "Rec_folder"() -> (w282:path)
                    n261 = Build Path(base path=w282, name or relative path="Info.txt") -> (appended path=w281:path)
                    n262 = Write to Text File(file (use dialog)=w281, text=w280) -> ()  [unwired: 2 in, 3 out]
                  }
                }
              }
              frame #7 {
                n263 = local write "Finished acquisition"(FALSE ("Finished acquisition")) -> ()
                n264 = local write "Acquire button"(FALSE ("Acquire button")) -> ()
                n265 = property on="Load settings" class="Bool (strict)"("DisabledEnum"=T6."Enabled" ("Disabled")) -> ()  [unwired: 2 in, 2 out]
                n266 = property on="Camera Control" class="Clust (strict)"("DisabledEnum"=T6."Enabled" ("Disabled")) -> ()  [unwired: 2 in, 2 out]
                n267 = property on="Focus button" class="Bool (strict)"("DisabledEnum"=T6."Enabled" ("Disabled")) -> ()  [unwired: 2 in, 2 out]
              }
            }
          }
          event "Camera Control": Value Change {
            # "Update camera settings"
            n268 = event-data() -> ()  [unwired: 1 in, 6 out]
            n269 = local read "Focus button"() -> (w290:bool)
            n270 = Not(x=w290) -> (.not. x?=w289:bool)
            n271 = case shown="True" w289 {
              frame False {
              }
              frame True {
                n272 = local read "Camera config"() -> (w299:string)
                n273 = local read "Camera Control"() -> (w301:T5)
                n274 = local read "Num frames"() -> (w296:u32)
                n275 = local read "Camera Session"() -> (w295:T1)
                n276 = local read "Camera Control"() -> (w297:T5)
                n277 = call "UpdateAllParameters.vi"("Camera Control"=w301, "Camera config in"=w299) -> ("Camera config out"=w298:string)
                n278 = call "AllocateImageBuffer.vi"("Camera Session"=w295, "Required num frames"=w296, "Camera Control"=w297) -> ("All Image Buffers"=w294:T4[], "#Frames Buffer"=w291:u32, "RAM Needed (GB)"=w293:dbl, "Recording Time (s)"=w292:dbl)
                n279 = local read "Camera Session"() -> (w300:T1)
                n280 = local write "Camera config"(w298) -> ()
                n281 = local write "All Image Buffers"(w294) -> ()
                n282 = local write "#Frames Buffer"(w291) -> ()
                n283 = local write "RAM needed (GB)"(w293) -> ()
                n284 = local write "Expected Time (s)"(w292) -> ()
                n285 = call <vilib>:"IMAQdx Read Attributes From String.vi"("Attributes String In"=w298, "Session In"=w300) -> ()  [unwired: 1 in, 9 out]
                n286 = property on="Buffer used (frames)" class="Slide (strict)"("Scale.Maximum"=w291) -> ()  [unwired: 2 in, 2 out]
              }
            }
          }
          event "Load settings": Value Change {
            n287 = event-data() -> ()  [unwired: 1 in, 6 out]
            n288 = stacked-sequence {
              frame #0 {
                # "Updating parameters and camera control"
                n289 = call "LoadParameters.vi"() -> ("Camera Control"=w303:T5, "Camera config"=w302:string)
                n290 = local write "Camera config"(w302) -> ()
                n291 = local write "Camera Control"(w303) -> ()
              }
              frame #1 {
                # "Updating the buffer"
                # "Wrting parameters into the camera"
                n292 = local read "Camera Control"() -> (w308:T5)
                n293 = local read "Num frames"() -> (w309:u32)
                n294 = local read "Camera Session"() -> (w310:T1)
                n295 = local read "Camera config"() -> (w311:string)
                n296 = local read "Camera Session"() -> (w312:T1)
                n297 = call "AllocateImageBuffer.vi"("Camera Session"=w310, "Required num frames"=w309, "Camera Control"=w308) -> ("All Image Buffers"=w307:T4[], "#Frames Buffer"=w304:u32, "RAM Needed (GB)"=w306:dbl, "Recording Time (s)"=w305:dbl)
                n298 = call <vilib>:"IMAQdx Read Attributes From String.vi"("Attributes String In"=w311, "Session In"=w312) -> ()  [unwired: 1 in, 9 out]
                n299 = local write "All Image Buffers"(w307) -> ()
                n300 = local write "#Frames Buffer"(w304) -> ()
                n301 = local write "RAM needed (GB)"(w306) -> ()
                n302 = local write "Expected Time (s)"(w305) -> ()
                n303 = property on="Buffer used (frames)" class="Slide (strict)"("Scale.Maximum"=w304) -> ()  [unwired: 2 in, 2 out]
              }
              frame #2 {
                n304 = local write "Load settings"(FALSE ("Load settings")) -> ()
              }
            }
          }
        }
      }
    }
  }
